vi "PCAN_CompMessage.vi"(1 "Detector2":bool, 2 "Detector1":bool, 3 "Excitation":bool) -> (0 "CAN_Message":T1)   [LabVIEW 2010]
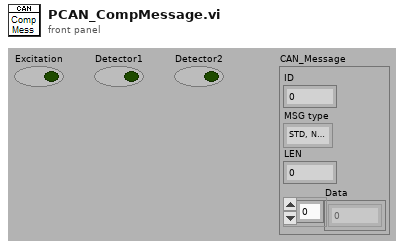
[diagram p1: front panel]
types:
  T1 = cluster{"ID":u32, "MSG type":enum8{"STD, NO RTR", "STD,RTR", "XTD, NO RTR", "XTD, RTR"}, "LEN":u8, "Data":u8[]}
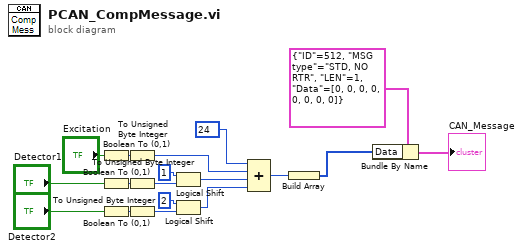
[diagram p0: block diagram]
diagram:
  n1 = Boolean To (0,1)(Boolean="Excitation") -> (0, 1=w4:i16)
  n2 = Boolean To (0,1)(Boolean="Detector1") -> (0, 1=w5:i16)
  n3 = Boolean To (0,1)(Boolean="Detector2") -> (0, 1=w7:i16)
  n4 = To Unsigned Byte Integer(number=w4) -> (unsigned 8bit integer=w15:u8)
  n5 = To Unsigned Byte Integer(number=w5) -> (unsigned 8bit integer=w9:u8)
  n6 = To Unsigned Byte Integer(number=w7) -> (unsigned 8bit integer=w11:u8)
  n7 = Logical Shift(y=i8 1, x=w9) -> (x << y=w13:u8)
  n8 = Logical Shift(y=i8 2, x=w11) -> (x << y=w14:u8)
  n9 = Compound Arithmetic op=ADD(u8 24 ("ID"), w15, w13, w14) -> (w16:u8)
  n10 = Build Array(w16) -> (w17:u8[])
  n11 = Bundle By Name(cluster=T1 {"ID"=512, "MSG type"=enum."STD, NO RTR", "LEN"=1, "Data"=[0, 0, 0, 0, 0, 0, 0, 0]} ("CAN_Message"), "Data"=w17) -> (→"CAN_Message":T1)
